vi "字符串过滤-域名.vi"(11 "字符串i":string) -> (0 "域名?":bool, 3 "字符串o":string)   [LabVIEW 2017]
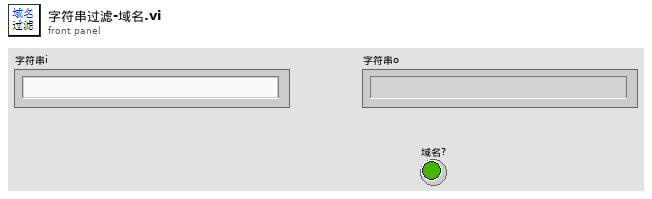
[diagram p1: front panel]
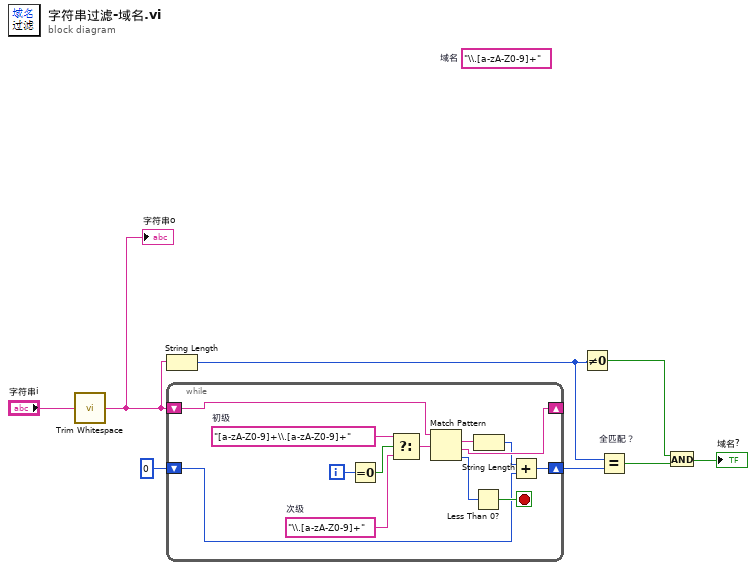
[diagram p0: block diagram]
diagram:
  (unwired) "\\.[a-zA-Z0-9]+"  # 域名
  n1 = call <vilib>:"Trim Whitespace.vi"("string"="字符串i") -> ("trimmed string"=w4:string)  [unwired: 1 in]
  "字符串o" <- w4
  n2 = String Length(string=w4) -> (length=w3:i32)
  n3 = while {
    shift-right: [w18] -> _
    shift-left: w4 -> [w21]
    shift-right: [w14] -> w7
    shift-left: 0 -> [w15]
    i -> [w13]
    stop <- w19 stop-if-true
    w10 = "\\.[a-zA-Z0-9]+"  # 次级
    w11 = "[a-zA-Z0-9]+\\.[a-zA-Z0-9]+"  # 初级
    n4 = Equal To 0?(x=w13) -> (x = 0?=w12:bool)
    n5 = Select(t=w11, s=w12, f=w10) -> (s? t:f=w9:string)
    n6 = Match Pattern(string=w21, regular expression=w9) -> (match substring=w17:string, after substring=w18:string, offset past match=w20:i32)  [unwired: 1 in, 1 out]
    n7 = Less Than 0?(x=w20) -> (x < 0?=w19:bool)
    n8 = String Length(string=w17) -> (length=w16:i32)
    n9 = Add(x=w16, y=w15) -> (x+y=w14:i32)
  }
  n10 = Not Equal To 0?(x=w3) -> (x != 0?=w1:bool)
  n11 = Equal? "全匹配？"(x=w3, y=w7) -> (x = y?=w6:bool)
  n12 = And(x=w1, y=w6) -> (x .and. y?=→"域名?":bool)
